vi "Heat Up Macro Measure 3 Min After.vi"(10 "Start Time":dbl, 11 "Array in":string[][](array[string])) -> (3 "Array out":string[][](array[string]))   [LabVIEW 2019]
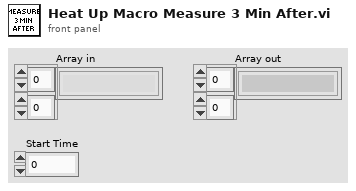
[diagram p1: front panel]
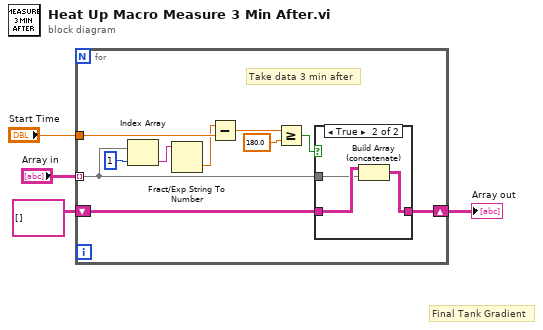
[diagram p0: block diagram]
diagram:
  # "Final Tank Gradient"
  n1 = for {
    tunnel: "Array in" -> [w8] mode=indexing
    tunnel: "Start Time" -> [w12]
    shift-right: [w7] -> w4
    shift-left: string[][] [] -> [w9]
    # "Take data 3 min after"
    n2 = Index Array(array=w8, index=1) -> (element=w13:string)
    n3 = Fract/Exp String To Number(string=w13) -> (number=w5:dbl)  [unwired: 3 in, 1 out]
    n4 = Subtract(x=w5, y=w12) -> (x-y=w6:dbl)
    n5 = Greater Or Equal?(x=w6, y=180.0) -> (x >= y?=w10:bool)
    n6 = case shown="True" w10 {
      tunnel: w9 -> [w15 w18]
      tunnel: w8 -> [_ w17]
      tunnel: [w15 w16] -> w7
      frame False {
      }
      frame True {
        n7 = Build Array (concatenate)(w18, w17) -> (w16:string[][])
      }
    }
  }
  "Array out" <- w4
